vi "QDInstrumentExceptionHandler.vi"(1 "Error in":errorcluster) -> (0 "Error out":errorcluster)   [LabVIEW 2019]
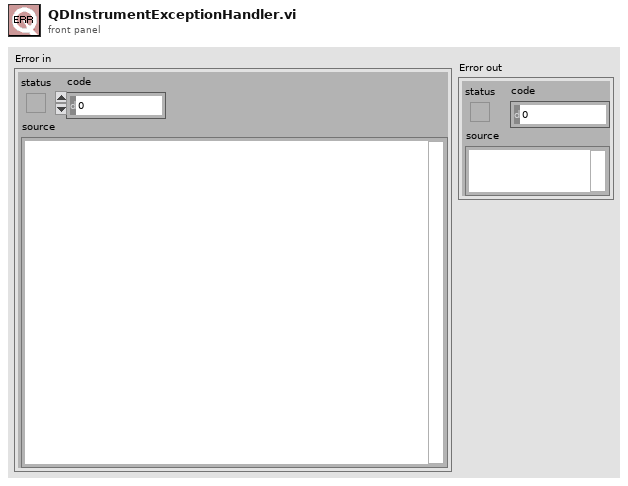
[diagram p1: front panel]
types:
  T1 = enum16{"Left Button", "Center Button", "Right Button", "Window Close"}
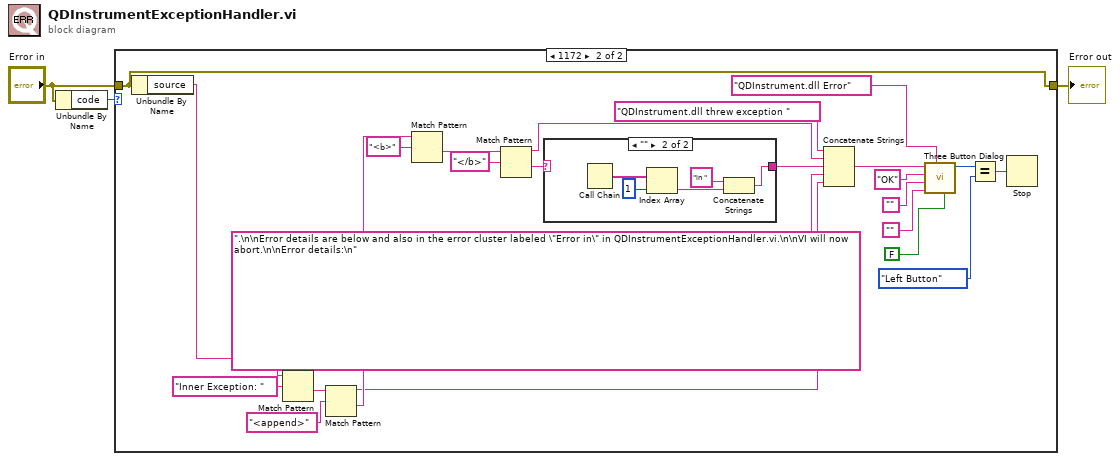
[diagram p0: block diagram]
diagram:
  n1 = Unbundle By Name("Error in") -> ("code"=w2:i32)
  n2 = case shown="1172" w2 {
    tunnel: "Error in" -> [w4 w21]
    tunnel: [w4 w21] -> w3
    frame 0, Default {
    }
    frame 1172 {
      n3 = Unbundle By Name(w21) -> ("source"=w18:string)
      n4 = Match Pattern(string=w18, regular expression="Inner Exception: ") -> (after substring=w16:string)  [unwired: 1 in, 3 out]
      n5 = Match Pattern(string=w16, regular expression="<append>") -> (before substring=w5:string, after substring=w14:string)  [unwired: 1 in, 2 out]
      n6 = Match Pattern(string=w14, regular expression="<b>") -> (after substring=w12:string)  [unwired: 1 in, 3 out]
      n7 = Match Pattern(string=w12, regular expression="</b>") -> (before substring=w9:string, after substring=w8:string)  [unwired: 1 in, 2 out]
      n8 = case shown="\"\"" w8 {
        selector: w8 -> [w29 _]
        tunnel: [w29 w30] -> w7
        frame "Not Blank", Default {
        }
        frame "" {
          n9 = Call Chain() -> (call chain=w33:string[])
          n10 = Index Array(array=w33, index=1) -> (element=w31:string)
          n11 = Concatenate Strings("in " ("string"), w31) -> (w30:string)
        }
      }
      n12 = Concatenate Strings("QDInstrument.dll threw exception " ("message"), w9, w7, ".\n\nError details are below and also in the error cluster labeled \"Error in\" in QDInstrumentExceptionHandler.vi.\n\nVI will now abort.\n\nError details:\n" ("string"), w5) -> (w27:string)
      n13 = call <vilib>:"Three Button Dialog.vi"("Allow user to close window? (TRUE)"=FALSE, "Window Title (\"\")"="QDInstrument.dll Error" ("Window Title (\"\")"), "Right Button Text (\"Cancel\")"="", "Center Button Text (\"No\")"="", "Left Button Text (\"Yes\")"="OK" ("Left Button Text (\"Yes\")"), "message"=w27) -> ("Which Button?"=w24:T1)  [unwired: 5 in]
      n14 = Equal?(x=w24, y=T1."Left Button") -> (x = y?=w22:bool)
      n15 = Stop(stop? (T)=w22) -> ()
    }
  }
  "Error out" <- w3
